vi "image-list--constant.vi"() -> (3 "image-list":path)   [LabVIEW 2021]
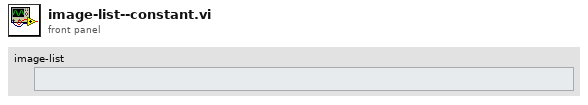
[diagram p1: front panel]
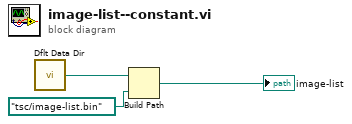
[diagram p0: block diagram]
diagram:
  n1 = call <vilib>:"Dflt Data Dir.vi"() -> ("App:Default Data Directory"=w1:path)
  n2 = Build Path(base path=w1, name or relative path=path "tsc/image-list.bin") -> (appended path=→"image-list":path)
